vi "about_dialog.vi"() -> ()   [LabVIEW 2010]
panel:
  in  "ok button":bool
  # "HelioScan"
  # "Concept and coordination: Dominik Langer\n\nImplementation: Dominik Langer, Marcel van 't Hoff, Thomasz Soltysinski, \nChetan Nagaraja, Maurice Göldi, Yves Kremer\n\nContact: langer@hifo.uzh.ch\n\nSee www.helioscan.org for details.\n\n© 2010 Helmchen Lab, Brain Research Institute, University of Zurich, Switzerland"
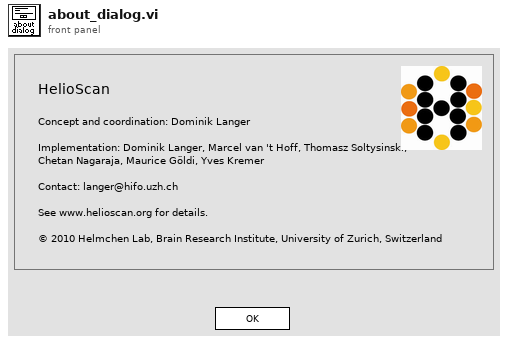
[diagram p1: front panel]
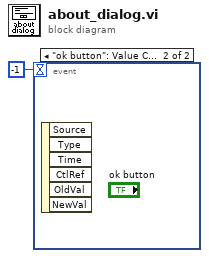
[diagram p0: block diagram]
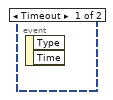
[diagram p2: hidden frame]
diagram:
  n1 = event shown="[1] \"ok button\": Value Change" {
    selector: _ -> [_ _]
    dyn-events: _ -> [_ _]
    timeout: -1 -> [_ _]
    event Timeout {
      n2 = event-data() -> ()  [unwired: 3 out]
    }
    event "ok button": Value Change {
      n3 = event-data() -> ()  [unwired: 7 out]
    }
  }
